vi "Initialize Daemon.vi"(8 "error in":errorcluster, 9 "Data Model":refnum<class "Device Data Model.lvclass">, 10 "transmission data unit":refnum<class "Transmission Data Unit.lvclass">, 11 "network slave in":refnum<class "Network Slave.lvclass">) -> (0 "error out":errorcluster, 3 "network slave out":refnum<class "Network Slave.lvclass">)   [LabVIEW 2012, in "Network Slave.lvclass"]
doc: "This provides an interface for the slave to launch a protocol daemon."
uses:
  Network Slave.lvclass
  Transmission Data Unit/Transmission Data Unit.lvclass
  Data Model/Device Data Model.lvclass
  daemon status cluster.ctl
  daemon status.ctl
  Network Slave.lvclass/Network Slave.ctl
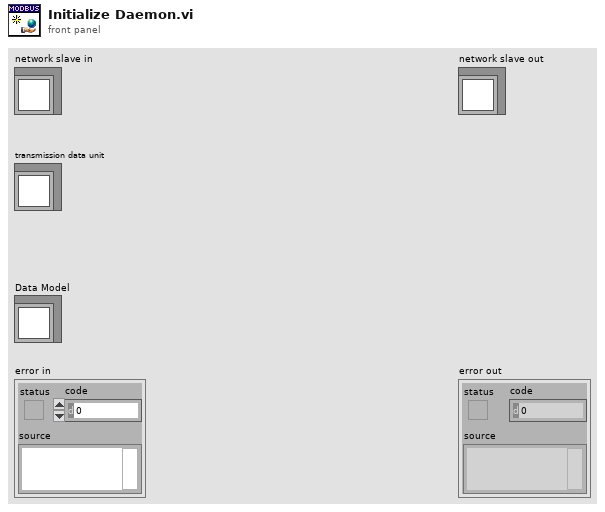
[diagram p1: front panel]
types:
  T1 = typedef "Network Slave.lvclass/daemon status cluster.ctl" = cluster{"error":errorcluster, "status":T2}
  T2 = typedef "Network Slave.lvclass/daemon status.ctl" = enum16{"Not Started", "Running", "Error", "Stopped"}
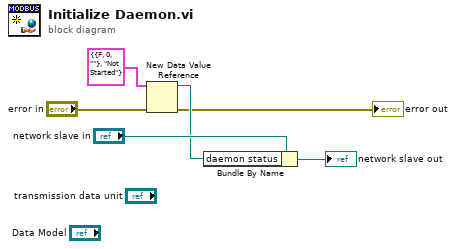
[diagram p0: block diagram]
diagram:
  n1 = New Data Value Reference(data value=T1 {"error"={"status"=FALSE, "code"=0, "source"=""}, "status"=enum."Not Started"} ("Status"), error in="error in") -> (data value reference=w3:refnum<data-value>, error out=→"error out":errorcluster)
  n2 = Bundle By Name(cluster="network slave in", "daemon status"=w3) -> (→"network slave out":refnum<class "Network Slave.lvclass">)
